vi "Web Service Error Handler.vi"(0 "LabVIEW Web Service Request":refnum<class "Web Request.lvclass">, 11 "error in (no error)":errorcluster) -> (4 "LabVIEW Web Service Request out":refnum<class "Web Request.lvclass">, 15 "error out":errorcluster)   [LabVIEW 2023]
doc: "Handles errors in an HTTP method VI by writing the error message to the client."
uses:
  <vilib>/wsapi/Web Request.lvclass
  <vilib>/Utility/error.llb/DialogType.ctl
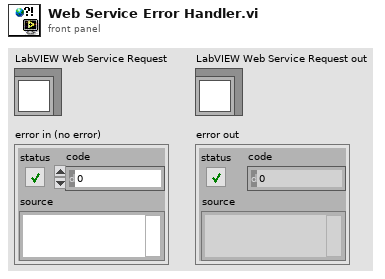
[diagram p1: front panel]
types:
  T1 = typedef "DialogType.ctl" = u16
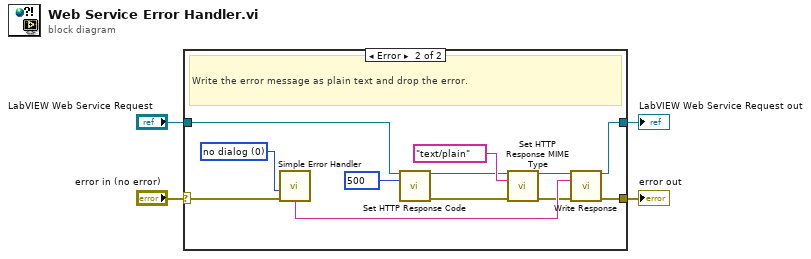
[diagram p0: block diagram]
diagram:
  n1 = case shown="Error" "error in (no error)" {
    selector: "error in (no error)" -> [w5 w14]
    tunnel: "LabVIEW Web Service Request" -> [w6 w9]
    tunnel: [w6 w16] -> w3
    tunnel: [w5 w15] -> w2
    frame No Error {
      # "Nothing to do when there is no error."
    }
    frame Error {
      w10 = 500 items=["100"=100, "101"=101, "200"=200, "201"=201, "202"=202, "203"=203, "204"=204, "205"=205, "206"=206, "300"=300, "301"=301, "302"=302, "303"=303, "304"=304, "305"=305, "306"=306, "307"=307, "400"=400, "401"=401, "402"=402, "403"=403, "404"=404, "405"=405, "406"=406, "407"=407, "408"=408, "409"=409, "410"=410, "411"=411, "412"=412, "413"=413, "414"=414, "415"=415, "416"=416, "417"=417, "500"=500, "501"=501, "502"=502, "503"=503, "504"=504, "505"=505] ("response code (200)")
      w17 = T1 0 items=["no dialog", "OK message", "continue or stop message", "OK message + warnings", "continue/stop + warnings"] ("type of dialog (OK msg:1)")
      # "Write the error message as plain text and drop the error."
      n2 = call <vilib>:"Simple Error Handler.vi"("type of dialog (OK msg:1)"=w17, "error in (no error)"=w14) -> ("message"=w18:string)  [unwired: 3 in, 4 out]
      n3 = call <vilib>:"Set HTTP Response Code.vi"("LabVIEW Web Service Request"=w9, "response code (200)"=w10) -> ("LabVIEW Web Service Request out"=w8:refnum<class "Web Request.lvclass">, "error out"=w11:errorcluster)  [unwired: 12 in]
      n4 = call <vilib>:"Set HTTP Response MIME Type.vi"("LabVIEW Web Service Request"=w8, "MIME type (text/html)"="text/plain", "error in (no error)"=w11) -> ("LabVIEW Web Service Request out"=w7:refnum<class "Web Request.lvclass">, "error out"=w13:errorcluster)  [unwired: 11 in]
      n5 = call <vilib>:"Write Response.vi"("LabVIEW Web Service Request"=w7, "response string"=w18, "error in (no error)"=w13) -> ("LabVIEW Web Service Request out"=w16:refnum<class "Web Request.lvclass">, "error out"=w15:errorcluster)  [unwired: 11 in]
    }
  }
  "LabVIEW Web Service Request out" <- w3
  "error out" <- w2
